vi "Process.vi"(0 "reference in":refnum<class "HPPC.lvclass">, 5 "error in":errorcluster) -> (14 "reference out":refnum<class "HPPC.lvclass">, 19 "error out":errorcluster)   [LabVIEW 2023, in "HPPC.lvclass"]
uses:
  HPPC.lvclass
  Types/DCIR Parameters.ctl
  Types/DCIR Mode.ctl
  Logger_class/Logger.lvclass
  <instrlib>/HPS-17000/HPS-17000.lvclass
  <vilib>/HPS-17000/nibatterycycler_grpc_Setpoint.ctl
  <vilib>/HPS-17000/Setpoint Stream Basic Config.ctl
  <vilib>/Utility/NIReport.llb/Report Type.ctl
  <instrlib>/HPS-17000/Internal/Set Energized Multi.vi
  <instrlib>/HPS-17000/Internal/Wait Until Energized Multi.vi
  <instrlib>/HPS-17000/Internal/Read Measurement Multi.vi
  <instrlib>/HPS-17000/Internal/Set Enabled Output Multi.vi
  <instrlib>/HPS-17000/Internal/Start Setpoint Stream Multi.vi
  <instrlib>/HPS-17000/Internal/Stream Setpoints Multi.vi
  <instrlib>/HPS-17000/Internal/Stop Setpoint Stream Multi.vi
  <instrlib>/HPS-17000/Internal/Write Setpoint Multi.vi
  <vilib>/printing/OpenHTMLReport.llb/Open HTML Report in Browser (Refnum).vi
  <vilib>/Utility/NIReport.llb/NI_report.lvclass
  HPPC.lvclass/HPPC.ctl
  <vilib>/Utility/SystemLogging/NI_SystemLogging.lvlib
  <vilib>/HPS-17000/NI_BC_client.lvlib
  <userlib>/_OpenG.lib/time/time.llb/openg_time.lvlib
  <vilib>/HPS-17000/Cycler.lvclass
  <vilib>/Utility/NIReport.llb/NI_ReportGenerationCore.lvlib
panel:
  out "Last Command":string
  out "error info":errorcluster
  in  "Save DCIR Report":bool
  in  "DCIR Tab Control":enum32{"PARAM", "PROFILE", "RUNNING", "NYQUIST"}(tab)
  out "DCIR Parameters":T1={"Initial SoC (%)"=650.0, "Pulse Mode"=2, "Pulse Current (A)"=1000.0, "Pulse Duration (S)"=500.0} {"Pulse Mode" items=["Discharge"=1, "Charge"=2]; "Initial SoC (%)" min=0.0 max=100.0}
  out "DCIR Profile":waveform(dbl)[](graph)
  out "Running Status Log":i32(listbox) caption="TEST SERVER LOG"
  out "DCIR Step":dbl[][](graph)
  out "DCIR Nyquist":cluster{dbl[], dbl[]}(graph)
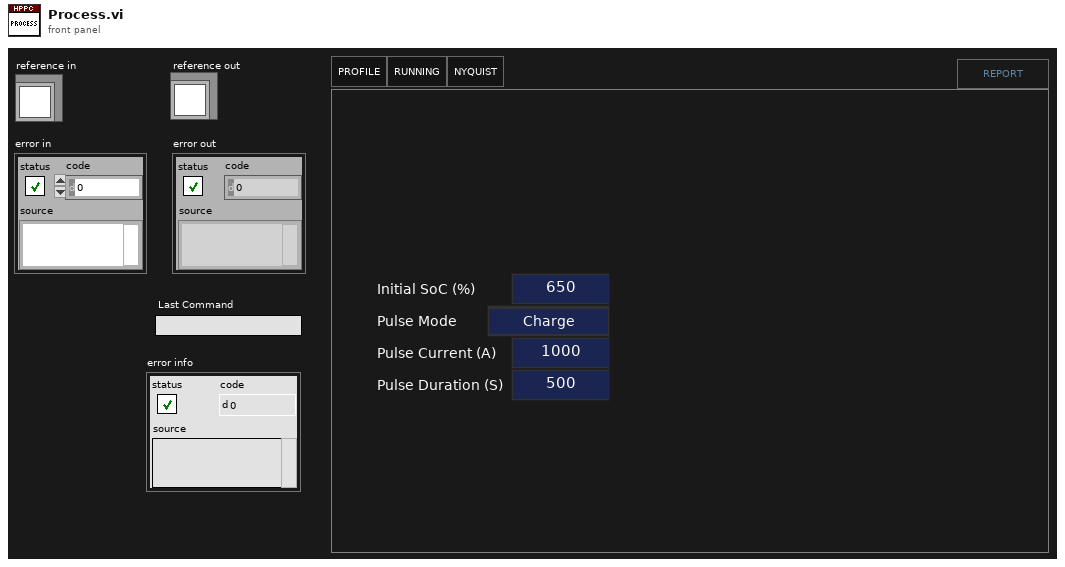
[diagram p1: front panel]
types:
  T1 = typedef "DCIR Parameters.ctl" = cluster{"Initial SoC (%)":dbl, "Pulse Mode":T2, "Pulse Current (A)":dbl, "Pulse Duration (S)":dbl}
  T2 = typedef "DCIR Mode.ctl" = u16
  T3 = cluster{"Core":cluster{"Timeout":i32, "Events":cluster{"EventsToProcess":refnum<event-registration>}, "EventFromProcess":refnum<user-event>, "ProcessSyncQueue":refnum<queue>, "QueueFromProcess":refnum<queue>, "Command":string, "Data":variant}, "DCIR Parameters":T1, "Profile Complete Event":refnum<user-event>, "DCIR Profile State":enum16{"Idle", "Start", "Run", "Stop"}, "DCIR TDMS Path":path, "Logger":refnum<class "Logger.lvclass">, "HPS17K Refs":refnum<class "HPS-17000.lvclass">[], "DCIR Profile":waveform(dbl)}
  T4 = typedef "Cycler.lvclass/Setpoint Stream Basic Config.ctl" = cluster{"local address":string, "receiver port":u16}
  T5 = typedef "NI_BC_client.lvlib/nibatterycycler_grpc_Setpoint.ctl" = cluster{"voltage":sgl, "current":sgl, "min_power":sgl, "max_power":sgl, "resistance":sgl}
  T6 = enum8{"Enabled", "Disabled", "Disabled and Grayed Out"}
  T7 = typedef "NI_ReportGenerationCore.lvlib/Report Type.ctl" = enum16{"HTML", "Word", "Excel"}
  T8 = enum32{"Invalid", "Standard", "Closed", "Hidden", "Minimized", "Maximized"}
  T9 = enum32{"PARAM", "PROFILE", "RUNNING", "NYQUIST", "PHASE", "MAGNITUDE"}
  T10 = cluster{"EventsToProcess":refnum<event-registration>}
  T11 = typedef "NI_BC_client.lvlib/MStream_grpc_CyclerMeasurement.ctl" = cluster{"measured_voltage":sgl, "measured_current":sgl, "setpoint_voltage":sgl, "setpoint_current":sgl, "timestamp":i64}
  T12 = typedef "HPPC.lvclass/ObjectAttributes.ctl" = cluster{"DCIR Parameters":T1, "Logger":refnum<class "Logger.lvclass">, "HPS17K Refs":refnum<class "HPS-17000.lvclass">[]}
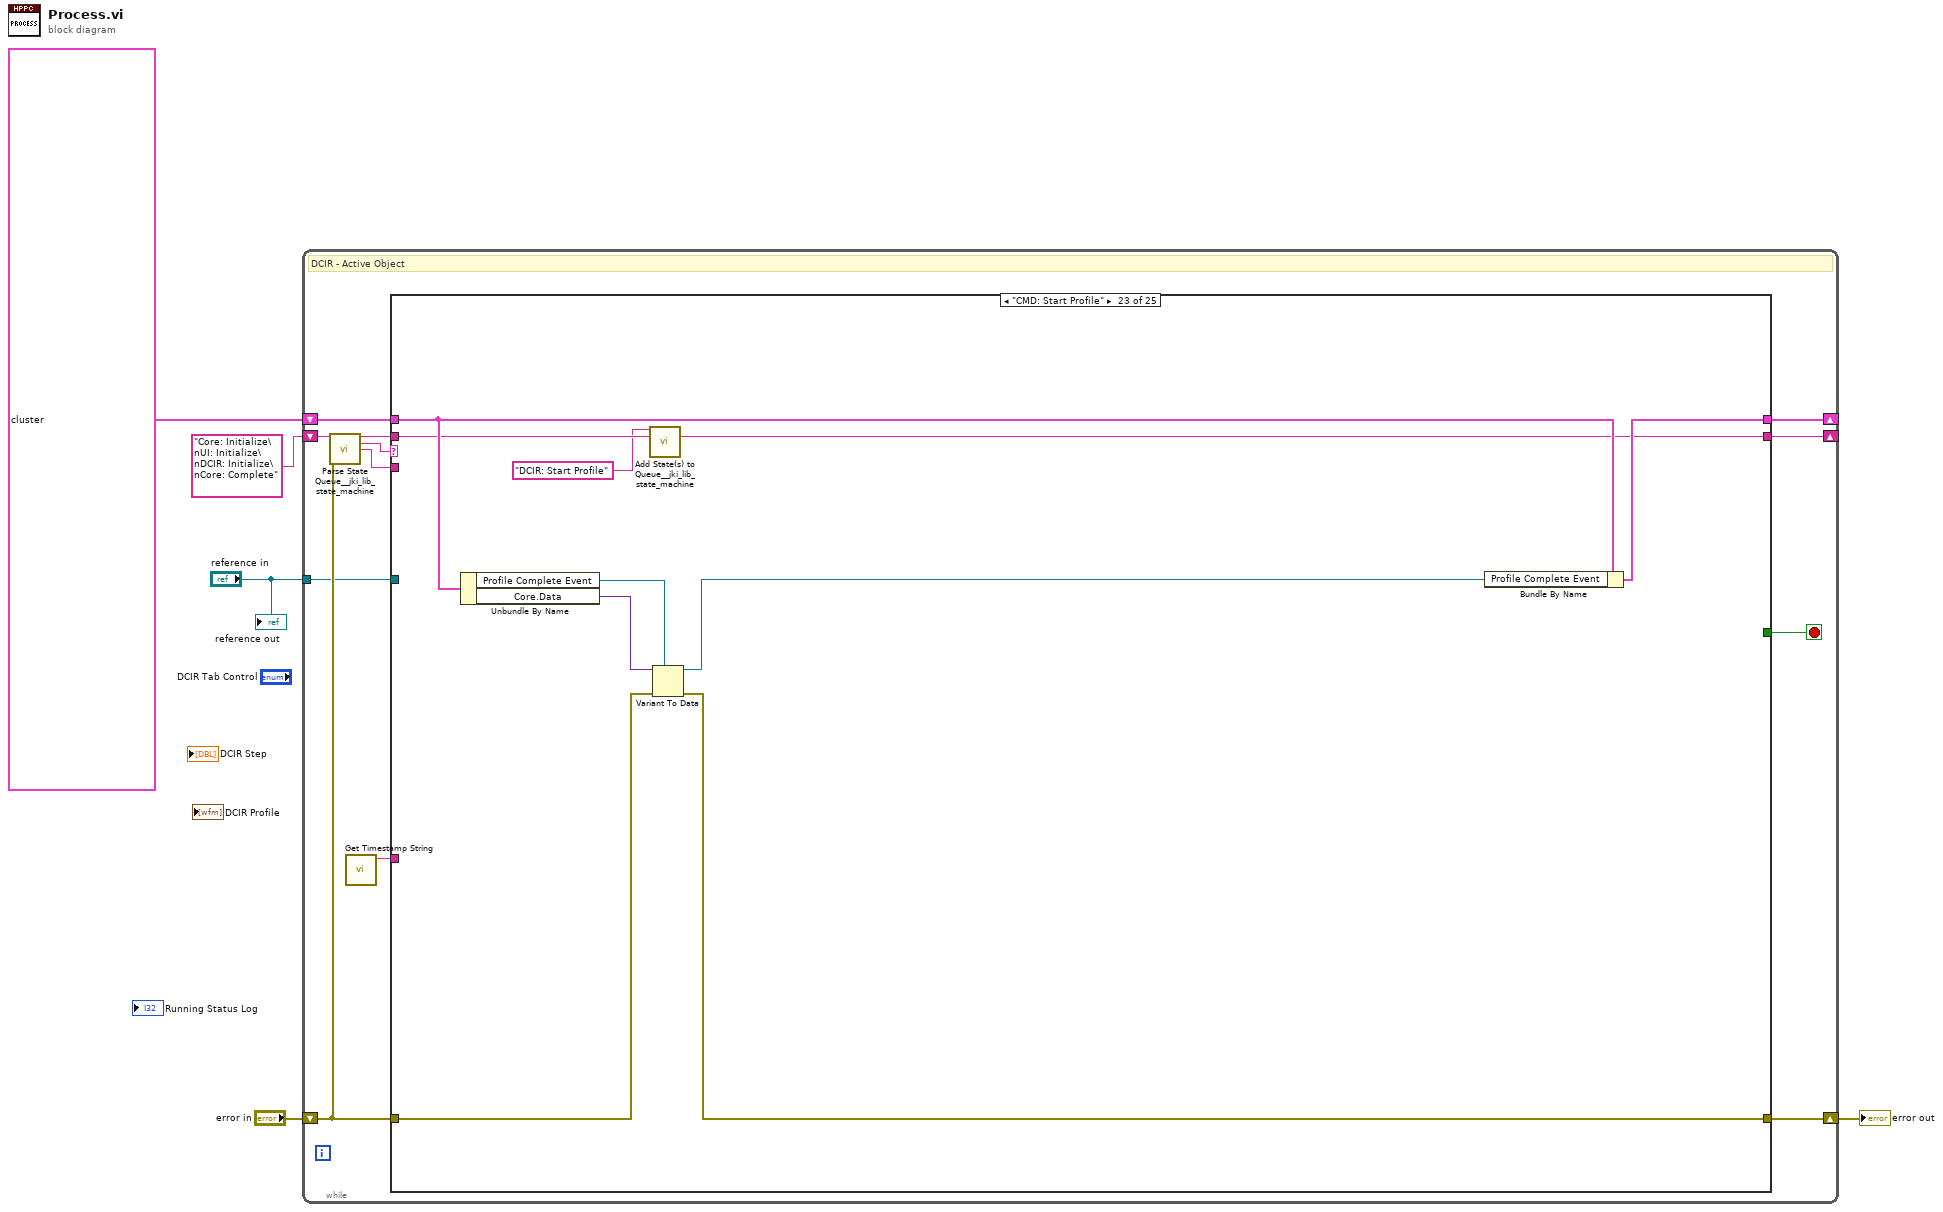
[diagram p0: block diagram]
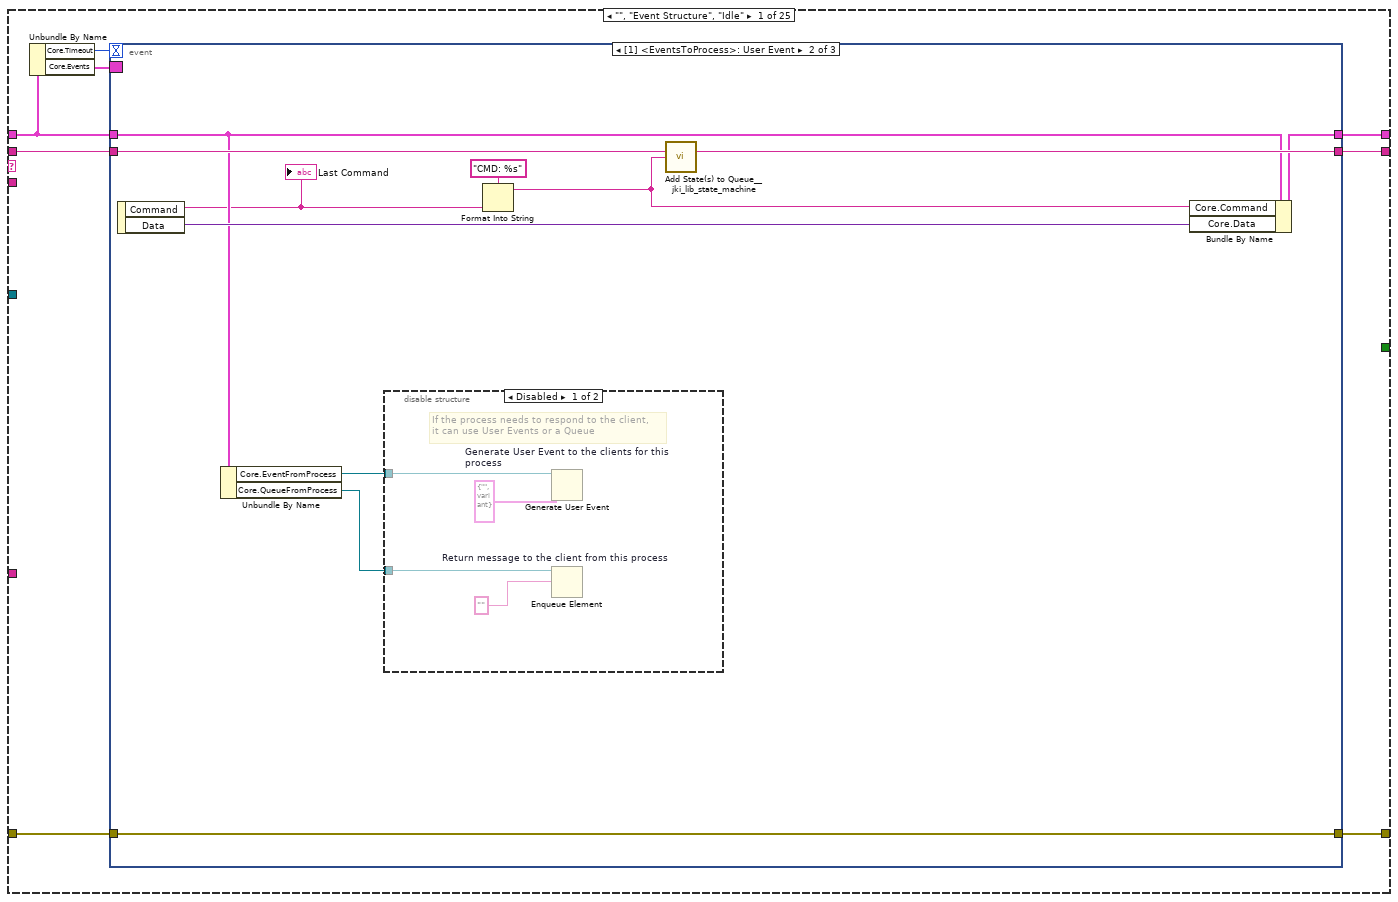
[diagram p2: hidden frame]
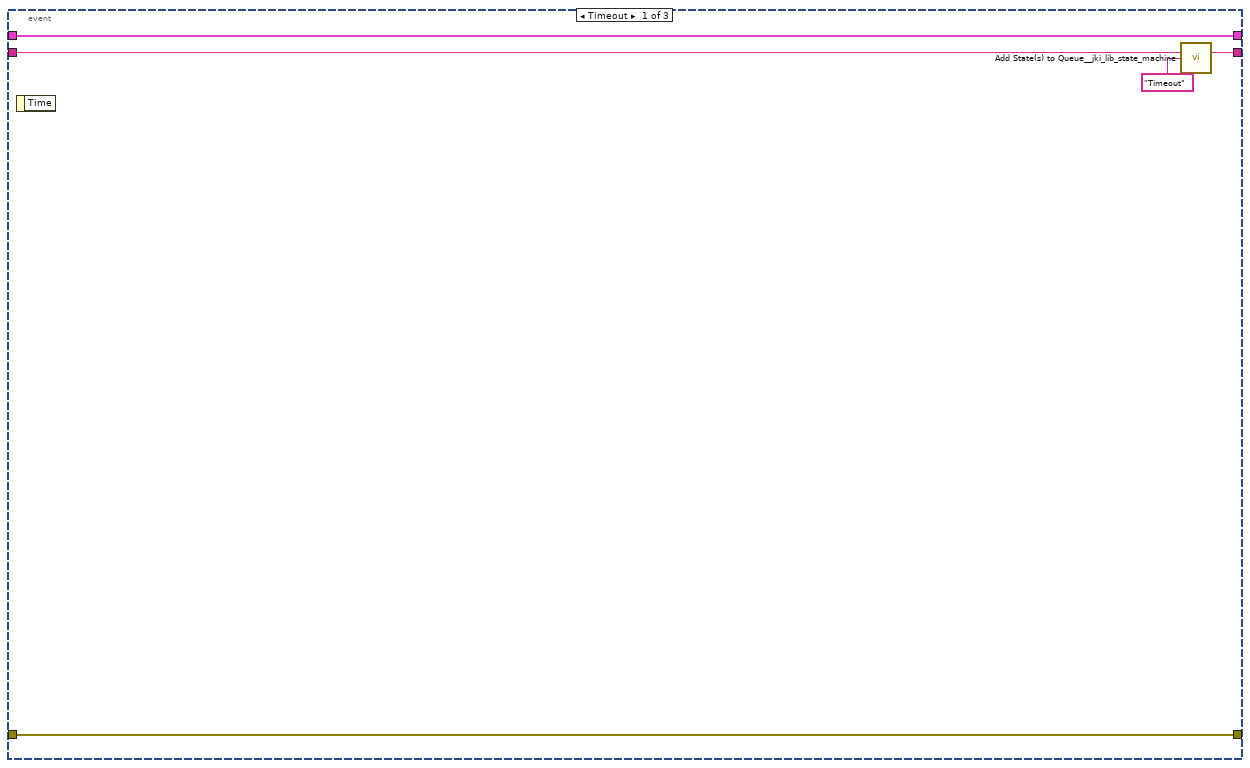
[diagram p3: hidden frame]
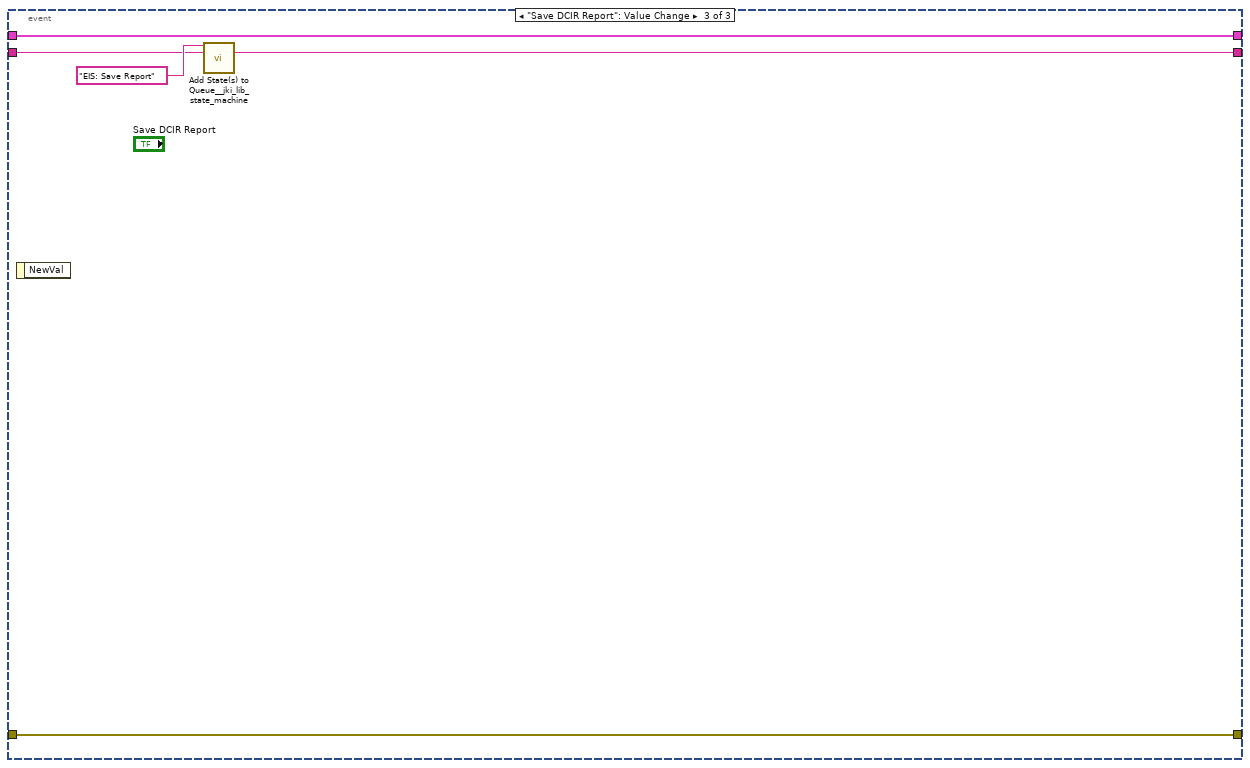
[diagram p5: hidden frame]
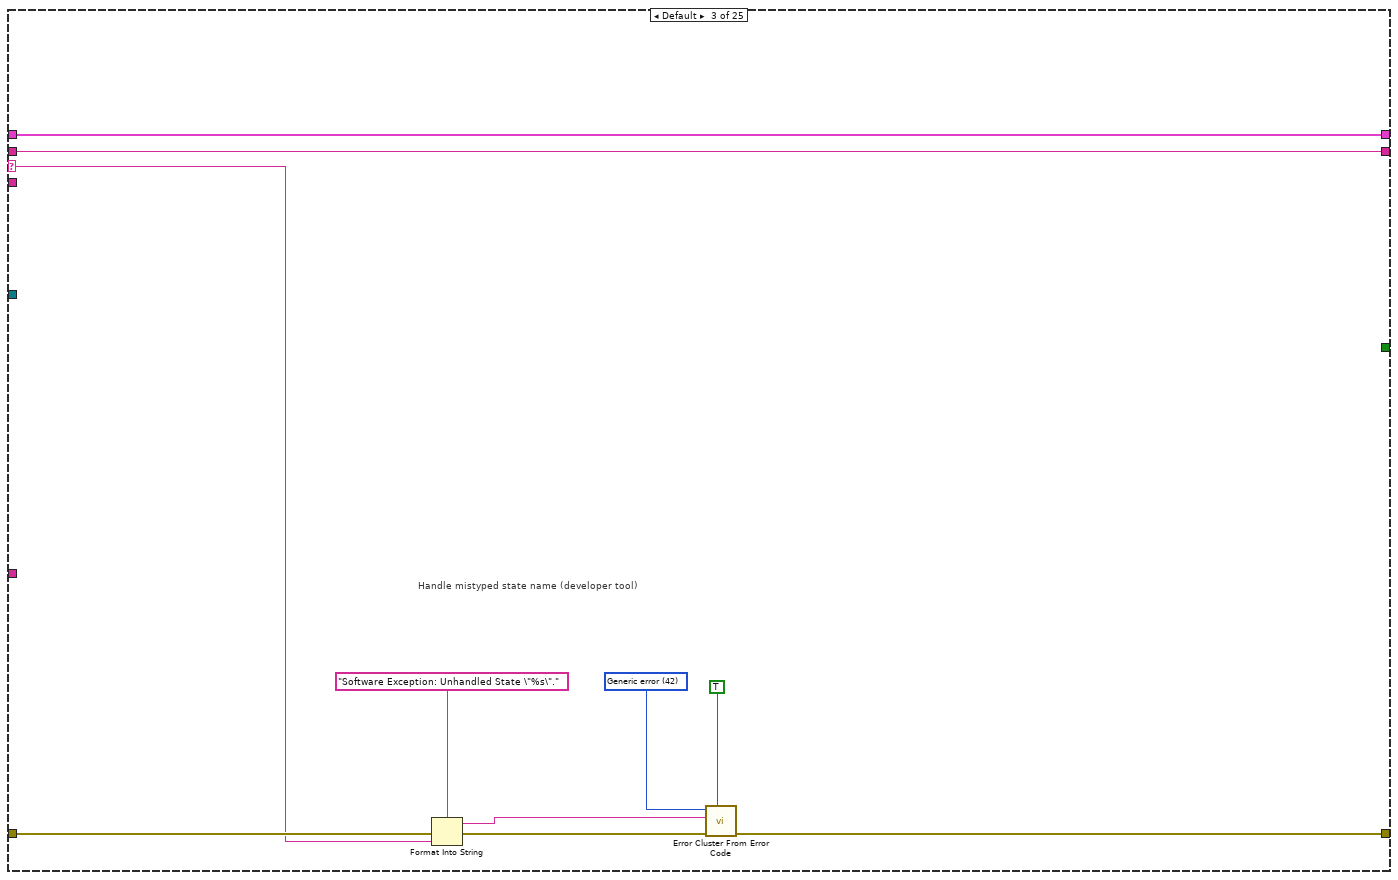
[diagram p7: hidden frame]
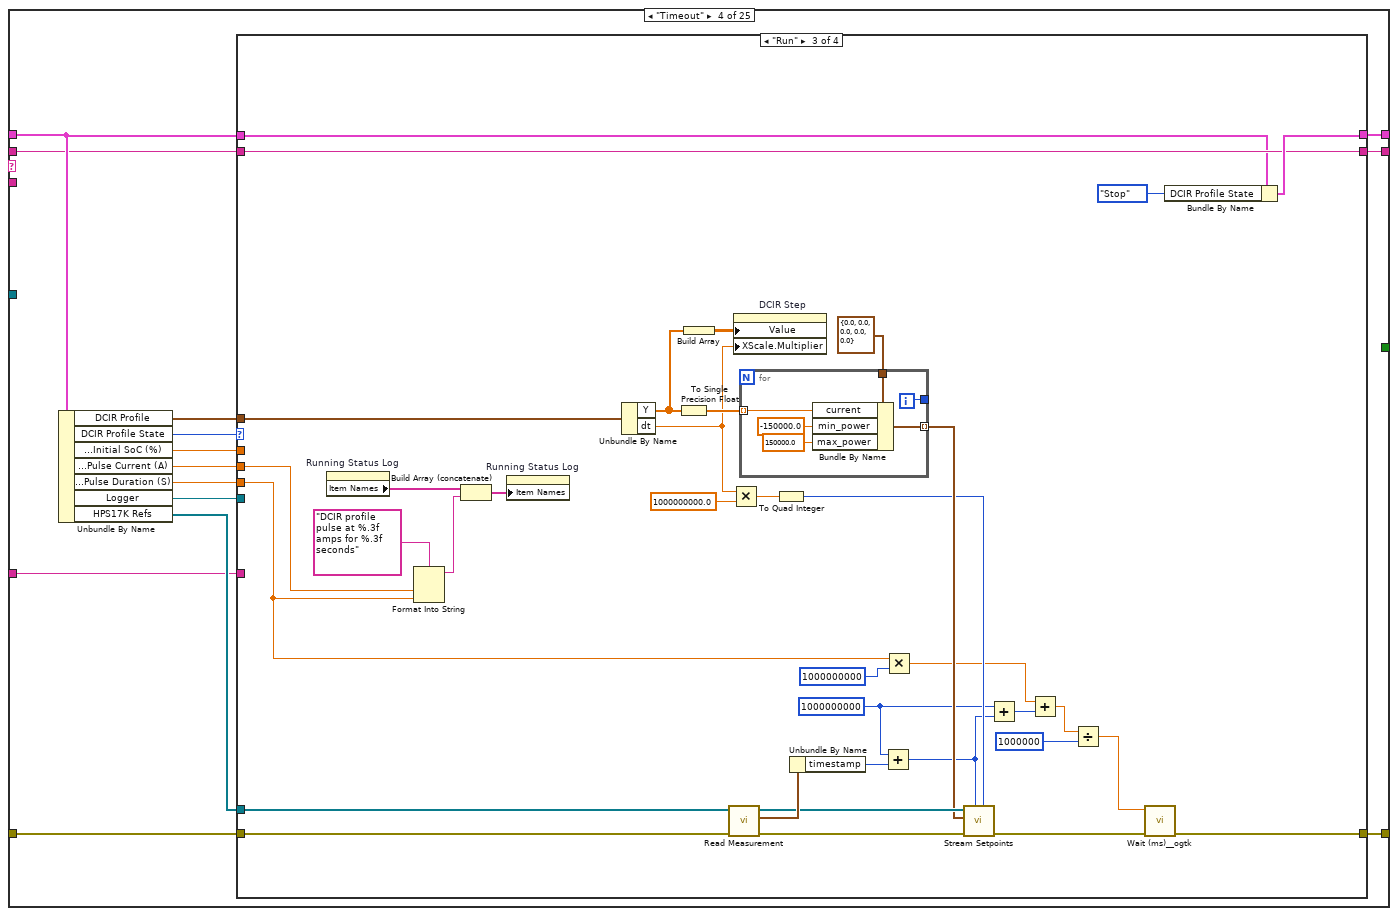
[diagram p8: hidden frame]
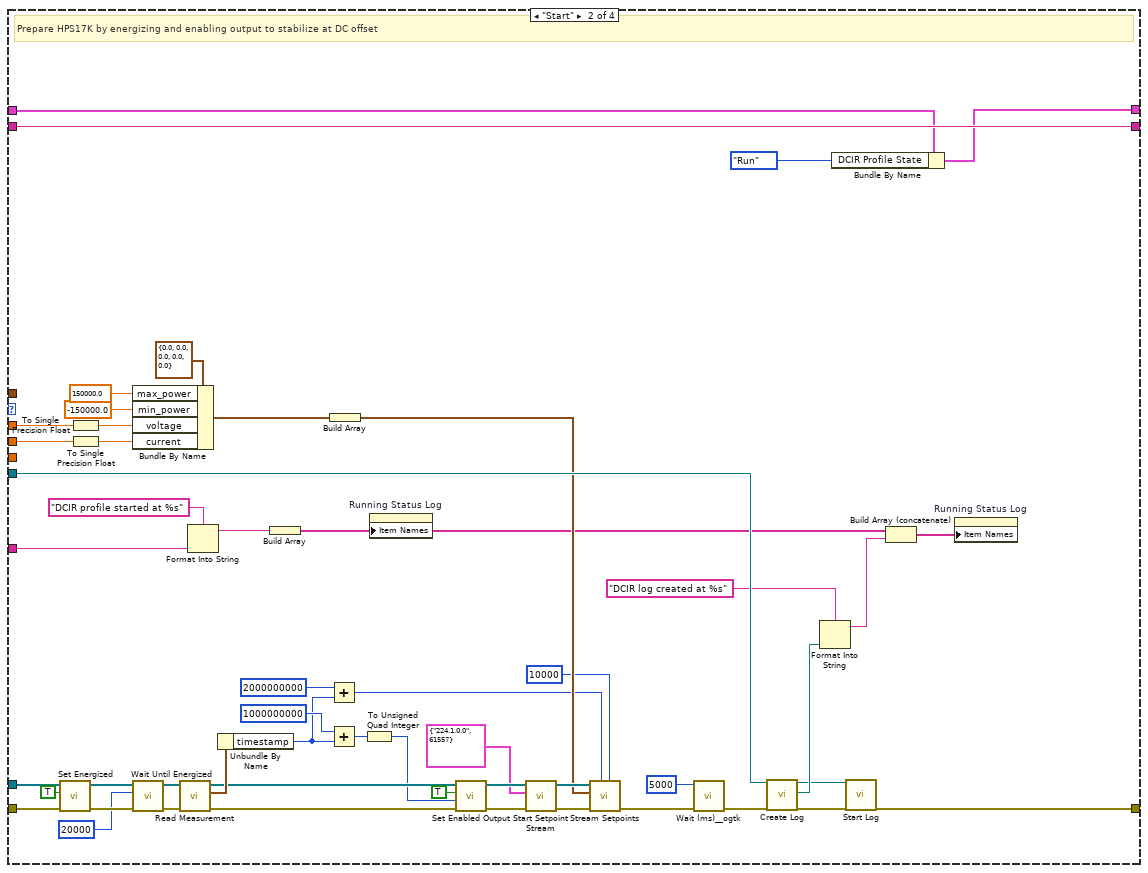
[diagram p10: hidden frame]
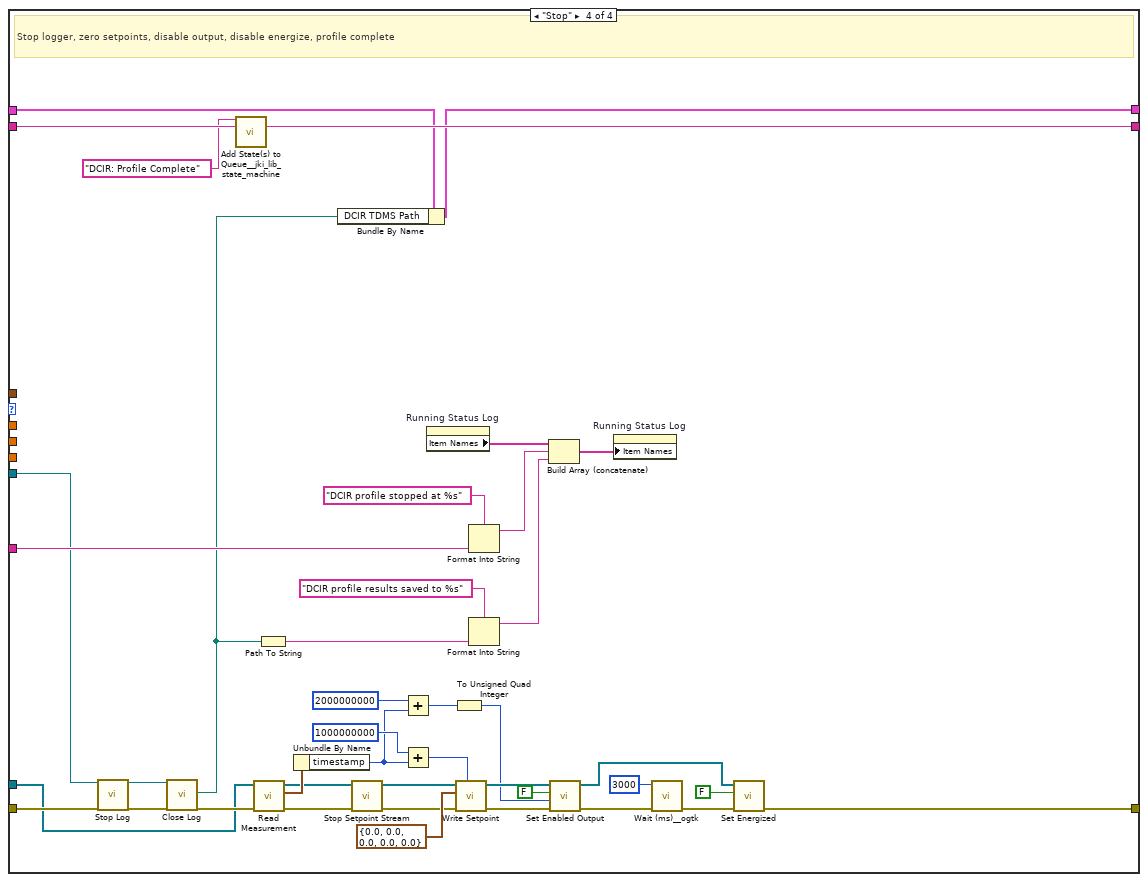
[diagram p11: hidden frame]
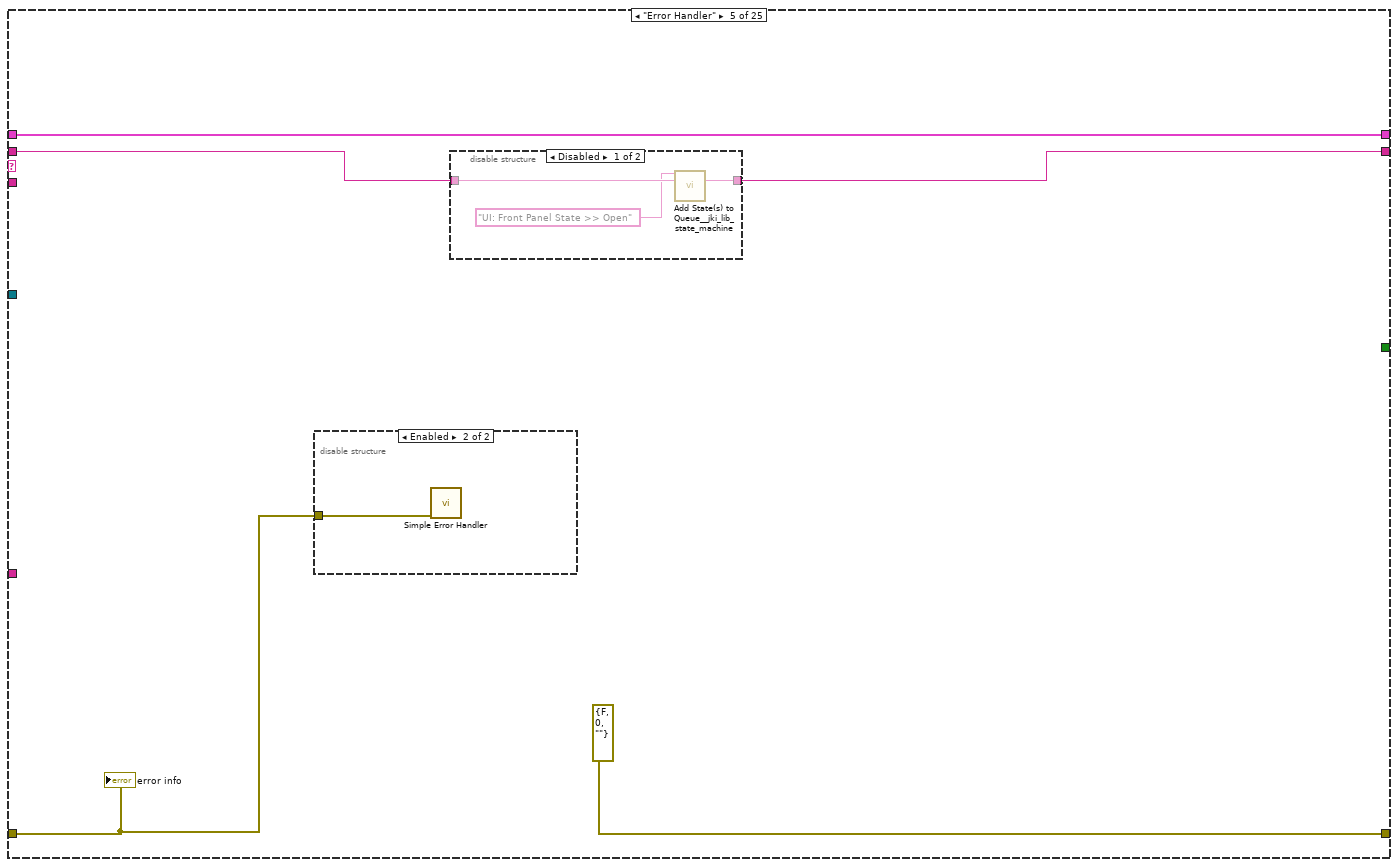
[diagram p12: hidden frame]
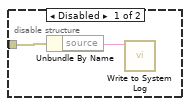
[diagram p14: hidden frame]
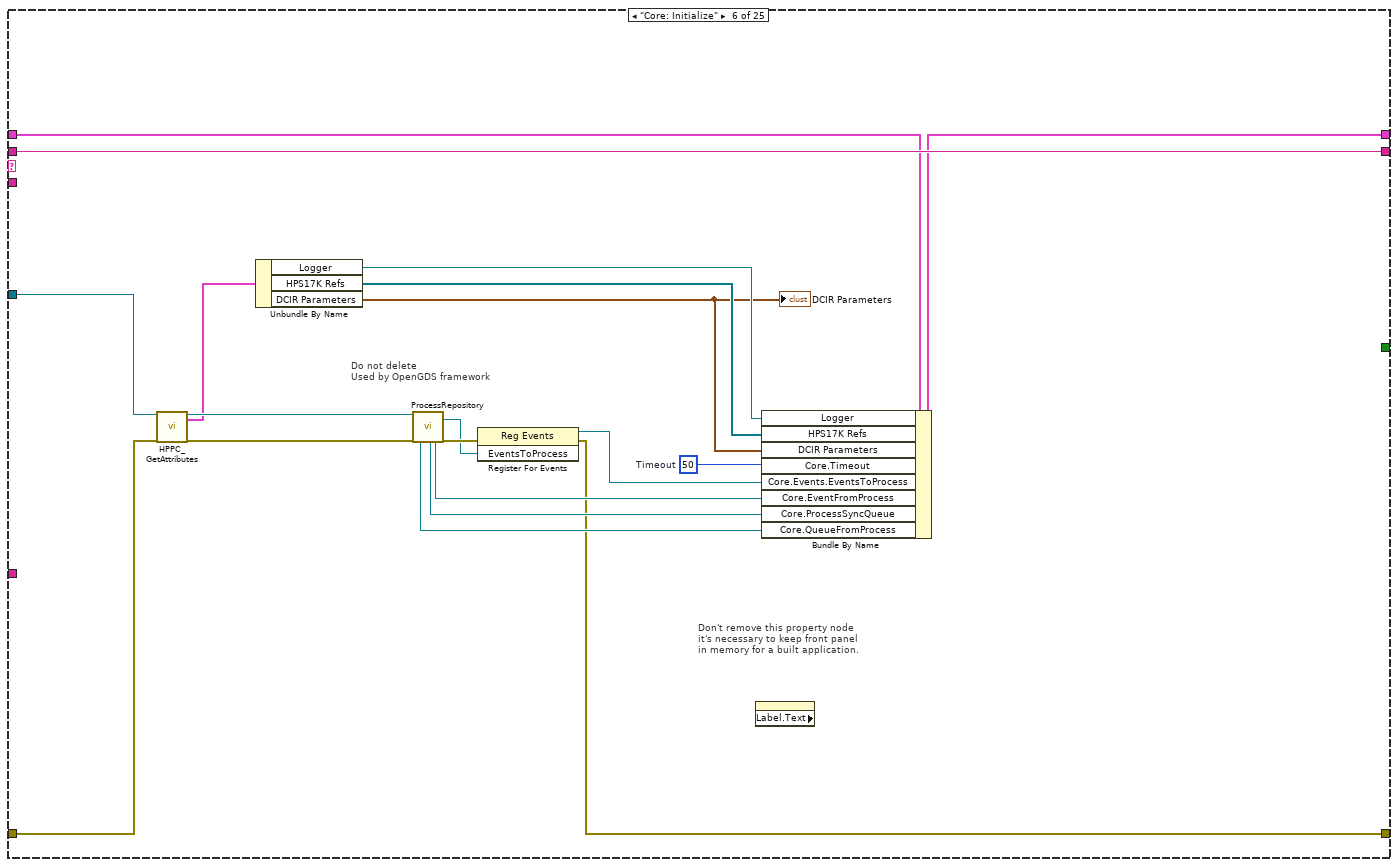
[diagram p15: hidden frame]
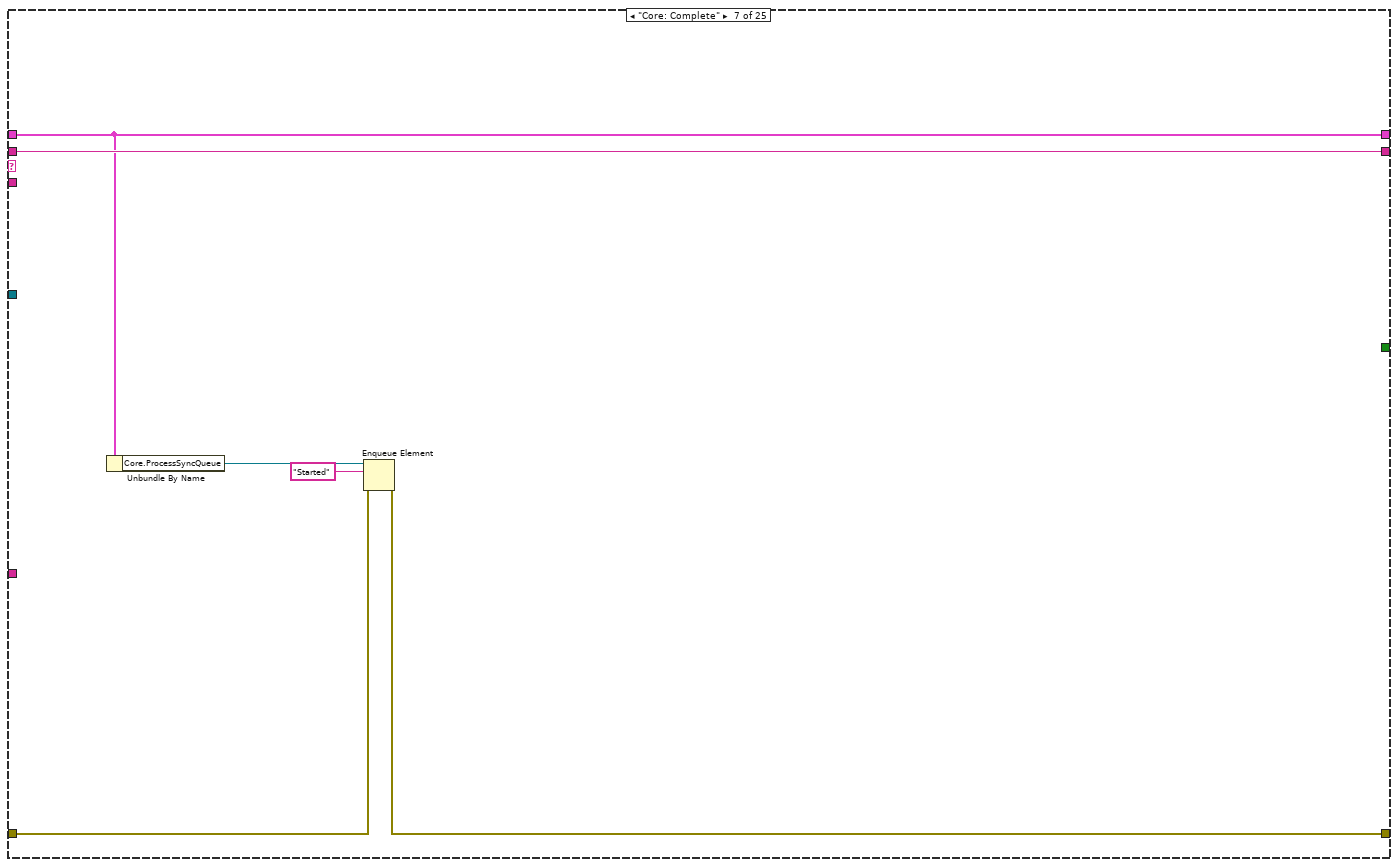
[diagram p16: hidden frame]
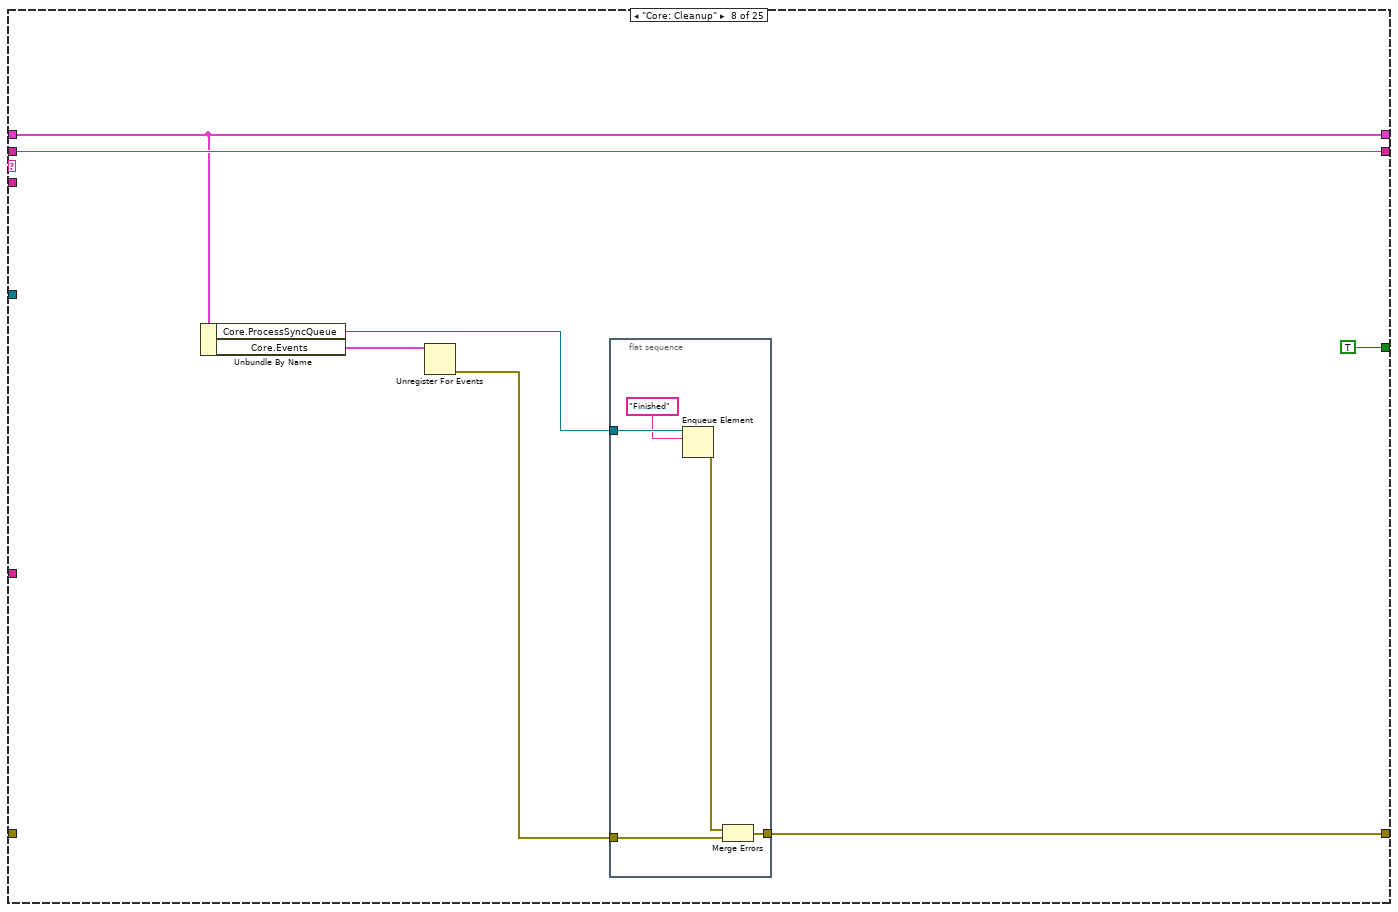
[diagram p17: hidden frame]
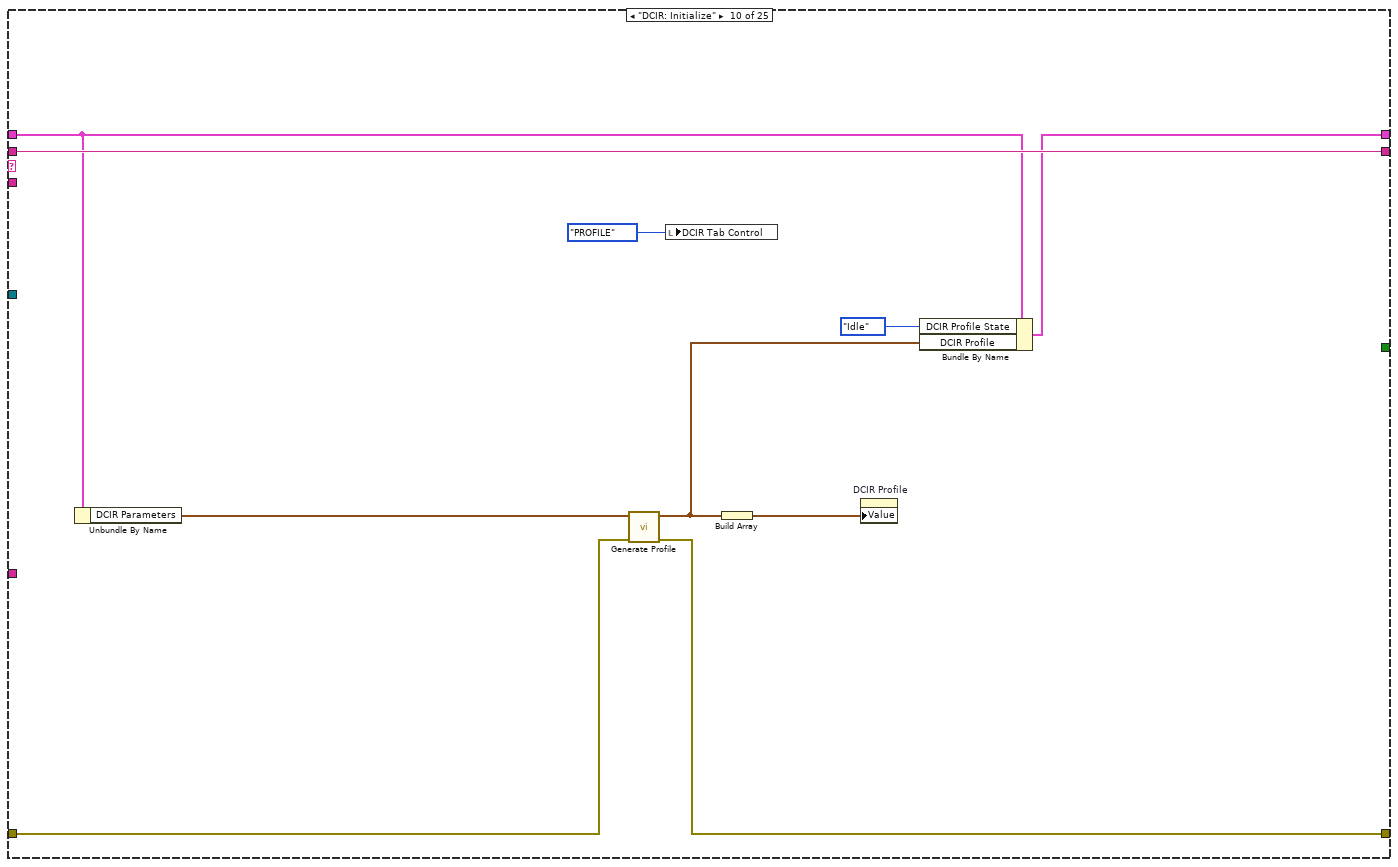
[diagram p19: hidden frame]
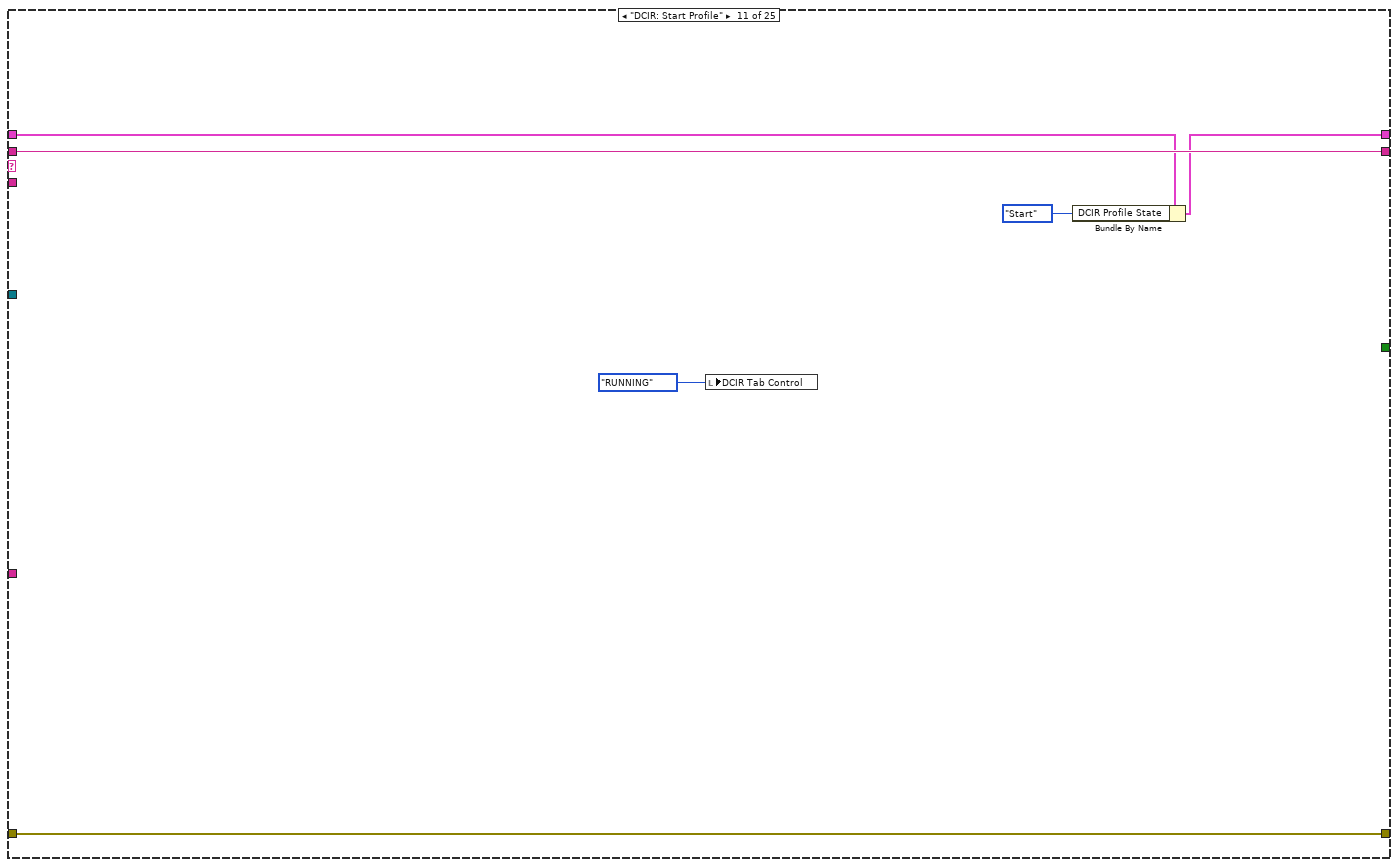
[diagram p20: hidden frame]
diagram:
  n1 = while {
    shift-right: [w16] -> w4
    shift-left: "error in" -> [w17]
    shift-right: [w9] -> _
    shift-left: "Core: Initialize\nUI: Initialize\nDCIR: Initialize\nCore: Complete" ("States Out") -> [w12]
    shift-right: [w15] -> _
    shift-left: T3 {"Core"={"Timeout"=-1, "Events"={"EventsToProcess"=refnum}, "EventFromProcess"=refnum, "ProcessSyncQueue"=refnum, "QueueFromProcess"=refnum, "Command"="", "Data"=variant}, "DCIR Parameters"={"Initial SoC (%)"=650.0, "Pulse Mode"=2, "Pulse Current (A)"=1000.0, "Pulse Duration (S)"=500.0}, "Profile Complete Event"=refnum, "DCIR Profile State"=enum."Idle", "DCIR TDMS Path"=path "", "Logger"=refnum, "HPS17K Refs"=[], "DCIR Profile"={"t0"=timestamp(0 s since 1904-01-01), "dt"=1.0, "Y"=[]}} ("LocalVariables") -> [w14]
    tunnel: "reference in" -> [w7]
    stop <- w8 stop-if-true
    # "DCIR - Active Object"
    n2 = call <vilib>:"Parse State Queue__jki_lib_state_machine.vi"("State Queue"=w12, "Error In (no error)"=w17) -> ("Remaining States"=w11:string, "Current State"=w13:string, "Arguments"=w10:string)  [unwired: 11 in]
    n3 = call "Get Timestamp String.vi"() -> ("date/time string"=w6:string)  [unwired: 11 in]
    n4 = case shown="\"CMD: Start Profile\"" w13 {
      selector: w13 -> [_ _ w54 _ _ _ _ _ _ _ _ _ _ _ _ _ _ _ _ _ _ _ _ _ _]
      tunnel: w17 -> [w19 w53 w56 w77 w217 w232 w248 _ w267 w276 w283 w288 w295 w305 w317 w364 w365 w393 _ w400 w403 w410 w418 w425 w430]
      tunnel: [w20 w53 w55 w76 errorcluster {"status"=FALSE, "code"=0, "source"=""} ("error constant") w237 w252 w255 w267 w275 w283 w288 w294 w303 w309 w364 w365 w393 w394 w400 w403 w410 w417 w425 w430] -> w16
      tunnel: [w25 w52 w63 w71 w220 w245 w249 w256 w266 w274 w280 w285 w292 w307 w319 w363 w367 w392 w395 w399 w402 w409 w415 w424 w429] -> w15
      tunnel: w14 -> [w21 w52 w63 w72 w220 w244 w249 w256 w266 w272 w281 w286 w293 w307 w319 w363 w367 w392 w395 w399 w402 w409 w416 w424 w429]
      tunnel: w11 -> [w23 w51 w62 w70 w219 w246 w251 w259 w265 w277 w282 w287 w299 w308 w318 w362 w368 w376 w397 w398 _ w408 w413 w423 w427]
      tunnel: w10 -> [_ _ _ _ _ _ _ _ _ _ _ _ _ _ _ _ w366 _ _ _ _ w405 _ _ _]
      tunnel: [w22 w51 w62 w69 w218 w246 w251 w259 w265 w277 w282 w287 w299 w308 w318 w362 w368 w376 w397 w398 "UI: Cleanup\nCore: Cleanup" ("State(s) at Back (\"\")") w407 w412 w422 w426] -> w9
      tunnel: [_ _ _ _ _ _ _ TRUE _ _ _ _ _ _ _ _ _ _ _ _ _ _ _ _ _] -> w8
      tunnel: w7 -> [_ _ _ _ _ w235 _ _ _ _ _ _ _ _ _ _ _ _ _ _ _ _ _ _ _]
      tunnel: w6 -> [_ _ _ w73 _ _ _ _ _ _ _ _ _ _ w311 _ _ _ _ _ _ _ _ _ _]
      frame "", "Event Structure", "Idle" {
        n5 = Unbundle By Name(w21) -> ("Core.Timeout"=w18:i32, "Core.Events"=w24:T10)
        n6 = event shown="[1] <EventsToProcess>: User Event" {
          selector: w24 -> [_ _ _]
          dyn-events: _ -> [_ _ _]
          timeout: w18 -> [_ _ _]
          tunnel: w21 -> [w30 w34 w50]
          tunnel: [w30 w39 w50] -> w25
          tunnel: [w28 w41 w46] -> w22
          tunnel: w23 -> [w29 w40 w47]
          tunnel: [w26 w35 w49] -> w20
          tunnel: w19 -> [w26 w35 w49]
          event Timeout {
            n7 = event-data() -> ()  [unwired: 1 in, 1 out]
            n8 = call <vilib>:"Add State(s) to Queue__jki_lib_state_machine.vi"("State(s) in (\"\")"=w29, "State(s) at Back (\"\")"="Timeout" ("State(s) at Back (\"\")")) -> ("States Out"=w28:string)  [unwired: 13 in]
          }
          event User Event {
            n9 = event-data() -> ("Command"=w32:string, "Data"=w38:variant)  [unwired: 1 in]
            "Last Command" <- w32
            n10 = Unbundle By Name(w34) -> ("Core.EventFromProcess"=w37:refnum<user-event>, "Core.QueueFromProcess"=w36:refnum<queue>)
            n11 = disable-structure shown="Disabled" {
              disable-tunnel: w37 -> [w45 _]
              disable-tunnel: w36 -> [w44 _]
              frame Disabled {
                # "If the process needs to respond to the client,\nit can use User Events or a Queue"
                n12 = Generate User Event "Generate User Event to the clients for this process"(user event=w45, event data cluster=cluster{"Command":string, "Data":variant} {"Command"="", "Data"=variant} ("event data")) -> ()  [unwired: 2 in, 2 out]
                n13 = Enqueue Element "Return message to the client from this process"(queue=w44, element="") -> ()  [unwired: 2 in, 3 out]
              }
              frame Enabled {
              }
            }
            n14 = Format Into String(format string="CMD: %s", w32) -> (resulting string=w31:string)  [unwired: 2 in, 1 out]
            n15 = call <vilib>:"Add State(s) to Queue__jki_lib_state_machine.vi"("State(s) in (\"\")"=w40, "State(s) at Back (\"\")"=w31) -> ("States Out"=w41:string)  [unwired: 13 in]
            n16 = Bundle By Name(cluster=w34, "Core.Command"=w31, "Core.Data"=w38) -> (w39:T3)
          }
          event "Save DCIR Report": Value Change {
            n17 = event-data() -> ()  [unwired: 1 in, 1 out]
            n18 = call <vilib>:"Add State(s) to Queue__jki_lib_state_machine.vi"("State(s) in Front (\"\")"="EIS: Save Report" ("State(s) in Front (\"\")"), "State(s) in (\"\")"=w47) -> ("States Out"=w46:string)  [unwired: 13 in]
          }
        }
      }
      frame "---------- Core ----------" {
      }
      frame Default {
        w60 = 42 items=["No error", "Argument error", "Memory is full", "Out of zone", "End of file", "File already open", "Generic file I/O error", "File not found", "File permission error", "Disk is full", "Duplicate path", "Too many files open", "System feature not enabled", "Resource file not found", "Cannot add resource", "Resource not found", "Image not found", "Image memory error", "Pen does not exist", "Config type invalid", "Config token not found", "Config parse error", "Config memory error", "Bad external code format", "Bad external code offset", "External code not present", "Null window", "Destroy window error", "Null menu", "Print aborted", "Bad print record", "Print driver error", "Windows error during printing", "Memory error during printing", "Print dialog error", "Generic print error", "Invalid device refnum", "Device not found", "Device parameter error", "Device unit error", "Cannot open device", "Device call aborted", "Generic error", "Cancelled by user", "Object ID too low", "Object ID too high", "Object not in heap", "Unknown heap", "Unknown object (invalid DefProc)", "Unknown object (DefProc not in table)", "Message out of range", "Invalid (null) method", "Unknown message", "Manager call not supported", "Bad address", "Network operation in progress", "Network operation timed out", "Connection is busy", "Network attribute not supported", "Network error", "Address in use", "System out of memory", "Connection aborted", "Connection refused", "Not connected", "Already connected", "Connection closed", "Initialization error (interapplication manager)", "Bad occurrence", "Wait on unbound occurrence handler", "Occurrence queue overflow", "Datalog type conflict", "Unused", "Unrecognized type (interapplication manager)", "Memory corrupt", "Failed to make temporary DLL", "Old CIN version", "Drag socket not found", "Failed to load drop-object", "Failed to register OLE object", "Failed to release OLE object", "Format specifier type mismatch", "Unknown format specifier", "Too few format specifiers", "Too many format specifiers", "Scan failed", "Newer CIN version", "Error converting to variant", "Runtime menu error", "Password tampered", "Variant attribute not found", "Incompatible variant data type", "Event data is not available", "Event Store is not present", "Occurrence is not found", "Event Queue is not created", "Event info is not available", "Refnum passed is NULL", "Error retrieving Class GUID", "Error retrieving CoClass GUID", "Error retrieving TypeLib GUID.", "Bad built application magic bytes.", "Specific driver is different from the specific driver associated with the Logical Name.", "There is no session opened to the class driver.", "Max Error", "MAX - Error with config objects", "MAX - Error loading configuration", "MAX - Group not supported"]
        # "Handle mistyped state name (developer tool)"
        n19 = Format Into String(format string="Software Exception: Unhandled State \"%s\"." ("message"), error in=w56, w54) -> (resulting string=w59:string, error out=w58:errorcluster)  [unwired: 1 in]
        n20 = call <vilib>:"Error Cluster From Error Code.vi"("show call chain? (False)"=TRUE, "error in (no error)"=w58, "error message (\"\")"=w59, "error code (0)"=w60) -> ("error out"=w55:errorcluster)  [unwired: 5 in]
      }
      frame "Timeout" {
        n21 = Unbundle By Name(w72) -> ("DCIR Profile"=w67:waveform(dbl), "DCIR Profile State"=w75:enum16{"Idle", "Start", "Run", "Stop"}, "DCIR Parameters.Initial SoC (%)"=w64:dbl, "DCIR Parameters.Pulse Current (A)"=w68:dbl, "DCIR Parameters.Pulse Duration (S)"=w65:dbl, "Logger"=w66:refnum<class "Logger.lvclass">, "HPS17K Refs"=w74:refnum<class "HPS-17000.lvclass">[])
        n22 = case shown="\"Run\"" w75 {
          tunnel: w77 -> [w80 w96 w167 w207]
          tunnel: [w80 w110 w146 w181] -> w76
          tunnel: w74 -> [_ w95 w166 w199]
          tunnel: w66 -> [_ w121 _ w204]
          tunnel: w73 -> [_ w116 _ w211]
          tunnel: w72 -> [w79 w106 w134 w180]
          tunnel: [w79 w105 w165 w179] -> w71
          tunnel: w70 -> [w78 w109 w164 w210]
          tunnel: [w78 w109 w164 w208] -> w69
          tunnel: w68 -> [_ w103 w148 _]
          tunnel: w64 -> [_ w102 _ _]
          tunnel: w67 -> [_ _ w149 _]
          tunnel: w65 -> [_ _ w137 _]
          frame "Idle", Default {
            # "do nothing"
          }
          frame "Start" {
            # "Prepare HPS17K by energizing and enabling output to stabilize at DC offset"
            n23 = call-poly <instrlib>:"Set Energized.vi"("error in"=w96, "energize (T)"=TRUE, "cycler refs in"=w95) -> ("error out"=w126:errorcluster, "cycler refs out"=w125:refnum<class "HPS-17000.lvclass">[])  [unwired: 7 in]
            n24 = To Single Precision Float(number=w102) -> (single precision float=w131:sgl)
            n25 = To Single Precision Float(number=w103) -> (single precision float=w128:sgl)
            n26 = Bundle By Name(cluster=T5 {"voltage"=0.0, "current"=0.0, "min_power"=0.0, "max_power"=0.0, "resistance"=0.0} ("setpoint"), "max_power"=sgl 150000.0, "min_power"=sgl -150000.0 ("max_power"), "voltage"=w131, "current"=w128) -> (w89:T5)
            n27 = call-poly <instrlib>:"Wait Until Energized.vi"("error in"=w126, "timeout (ms)"=u32 20000, "cycler refs in"=w125) -> ("error out"=w94:errorcluster, "cycler refs out"=w93:refnum<class "HPS-17000.lvclass">[])  [unwired: 7 in]
            n28 = call-poly <instrlib>:"Read Measurement.vi"("error in"=w94, "cycler refs in"=w93) -> ("error out"=w92:errorcluster, "aggregated cycler measurements"=w127:T11, "cycler refs out"=w91:refnum<class "HPS-17000.lvclass">[])  [unwired: 7 in]
            n29 = Format Into String(format string="DCIR profile started at %s", w116) -> (resulting string=w82:string)  [unwired: 2 in, 1 out]
            n30 = Unbundle By Name(w127) -> ("timestamp"=w97:i64)
            n31 = Build Array(w82) -> (w81:string[])
            n32 = Add(x=i64 2000000000, y=w97) -> (x+y=w86:i64)
            n33 = Add(x=i64 1000000000, y=w97) -> (x+y=w87:i64)
            n34 = Build Array(w89) -> (w88:T5[])
            n35 = To Unsigned Quad Integer(1:w87) -> (0:w85:u64)
            n36 = property on="Running Status Log" class="LstBox (strict)"("Item Names"=w81) -> ()  [unwired: 2 in, 2 out]
            n37 = call-poly <instrlib>:"Set Enabled Output.vi"("error in"=w92, "enabled timestamp"=w85, "enabled output"=TRUE, "cycler refs in"=w91) -> ("error out"=w101:errorcluster, "cycler refs out"=w100:refnum<class "HPS-17000.lvclass">[])  [unwired: 6 in]
            n38 = call-poly <instrlib>:"Start Setpoint Stream.vi"("error in"=w101, "setpoint stream config"=T4 {"local address"="224.1.0.0", "receiver port"=61557}, "cycler refs in"=w100) -> ("error out"=w98:errorcluster, "cycler refs out"=w90:refnum<class "HPS-17000.lvclass">[])  [unwired: 7 in]
            n39 = call-poly <instrlib>:"Stream Setpoints.vi"("dt"=i64 10000, "t0"=w86, "error in"=w98, "setpoints"=w88, "cycler refs in"=w90) -> ("error out"=w84:errorcluster)  [unwired: 5 in, 1 out]
            n40 = call <userlib>:"Wait (ms)__ogtk.vi"("error in (no error)"=w84, "milliseconds to wait"=u32 5000) -> ("error out"=w120:errorcluster)  [unwired: 8 in, 1 out]
            n41 = call "Create Log.vi"("reference in"=w121, "Error In"=w120) -> ("reference out"=w113:refnum<class "Logger.lvclass">, "created file"=w114:path, "Error Out"=w118:errorcluster)  [unwired: 15 in]
            n42 = Format Into String(format string="DCIR log created at %s", w114) -> (resulting string=w112:string)  [unwired: 2 in, 1 out]
            n43 = Bundle By Name(cluster=w106, "DCIR Profile State"=enum16{"Idle", "Start", "Run", "Stop"}."Run" ("EIS Profile State")) -> (w105:T3)
            n44 = call "Start Log.vi"("reference in"=w113, "Error In"=w118) -> ("Error Out"=w110:errorcluster)  [unwired: 16 in, 1 out]
            n45 = Build Array (concatenate)(w81, w112) -> (w111:string[])
            n46 = property on="Running Status Log" class="LstBox (strict)"("Item Names"=w111) -> ()  [unwired: 2 in, 2 out]
          }
          frame "Run" {
            w143 = i64 1000000000 ("x")
            n47 = property on="Running Status Log" class="LstBox (strict)"() -> ("Item Names"=w161:string[])  [unwired: 2 in, 2 out]
            n48 = Format Into String(format string="DCIR profile pulse at %.3f amps for %.3f seconds", w148, w137) -> (resulting string=w158:string)  [unwired: 2 in, 1 out]
            n49 = Build Array (concatenate)(w161, w158) -> (w157:string[])
            n50 = property on="Running Status Log" class="LstBox (strict)"("Item Names"=w157) -> ()  [unwired: 2 in, 2 out]
            n51 = Unbundle By Name(w149) -> ("Y"=w155:dbl[], "dt"=w150:dbl)
            n52 = To Single Precision Float(number=w155) -> (single precision float=w159:sgl[])
            n53 = Build Array(w155) -> (w135:dbl[][])
            n54 = call-poly <instrlib>:"Read Measurement.vi"("error in"=w167, "cycler refs in"=w166) -> ("error out"=w163:errorcluster, "aggregated cycler measurements"=w168:T11, "cycler refs out"=w162:refnum<class "HPS-17000.lvclass">[])  [unwired: 7 in]
            n55 = Multiply(x=w150, y=1000000000.0) -> (x*y=w153:dbl)
            n56 = property on="DCIR Step" class="WFGraph (strict)"("Value"=w135, "XScale.Multiplier"=w150) -> ()  [unwired: 2 in, 2 out]
            n57 = for {
              tunnel: T5 {"voltage"=0.0, "current"=0.0, "min_power"=0.0, "max_power"=0.0, "resistance"=0.0} ("nibatterycycler_grpc_Setpoint") -> [w174]
              tunnel: w159 -> [w173] mode=indexing
              tunnel: [w170] -> w152 mode=indexing
              tunnel: [w169] -> _
              i -> [w169]
              n58 = Bundle By Name(cluster=w174, "current"=w173, "min_power"=sgl -150000.0, "max_power"=sgl 150000.0) -> (w170:T5)
            }
            n59 = To Quad Integer(1:w153) -> (0:w151:i64)
            n60 = Unbundle By Name(w168) -> ("timestamp"=w133:i64)
            n61 = Add(x=w143, y=w133) -> (x+y=w144:i64)
            n62 = Multiply(x=w137, y=i64 1000000000 ("x")) -> (x*y=w136:dbl)
            n63 = call-poly <instrlib>:"Stream Setpoints.vi"("dt"=w151, "t0"=w144, "error in"=w163, "setpoints"=w152, "cycler refs in"=w162) -> ("error out"=w147:errorcluster)  [unwired: 5 in, 1 out]
            n64 = Add(x=w143, y=w144) -> (x+y=w142:i64)
            n65 = Add(x=w136, y=w142) -> (x+y=w141:dbl)
            n66 = Divide(x=w141, y=i64 1000000 ("x")) -> (x/y=w139:dbl)
            n67 = call <userlib>:"Wait (ms)__ogtk.vi"("error in (no error)"=w147, "milliseconds to wait"=w139) -> ("error out"=w146:errorcluster)  [unwired: 8 in, 1 out]
            n68 = Bundle By Name(cluster=w134, "DCIR Profile State"=enum16{"Idle", "Start", "Run", "Stop"}."Stop") -> (w165:T3)
          }
          frame "Stop" {
            # "Stop logger, zero setpoints, disable output, disable energize, profile complete"
            n69 = call "Stop Log.vi"("reference in"=w204, "Error In"=w207) -> ("reference out"=w205:refnum<class "Logger.lvclass">, "Error Out"=w206:errorcluster)  [unwired: 16 in]
            n70 = call "Close Log.vi"("reference in"=w205, "Error In"=w206) -> ("log file path"=w175:path, "Error Out"=w200:errorcluster)  [unwired: 15 in, 1 out]
            n71 = call <vilib>:"Add State(s) to Queue__jki_lib_state_machine.vi"("State(s) in Front (\"\")"="DCIR: Profile Complete" ("State(s) in Front (\"\")"), "State(s) in (\"\")"=w210) -> ("States Out"=w208:string)  [unwired: 13 in]
            n72 = call-poly <instrlib>:"Read Measurement.vi"("error in"=w200, "cycler refs in"=w199) -> ("error out"=w185:errorcluster, "aggregated cycler measurements"=w203:T11, "cycler refs out"=w184:refnum<class "HPS-17000.lvclass">[])  [unwired: 7 in]
            n73 = Path To String(path=w175) -> (string=w177:string)
            n74 = Unbundle By Name(w203) -> ("timestamp"=w194:i64)
            n75 = Bundle By Name(cluster=w180, "DCIR TDMS Path"=w175) -> (w179:T3)
            n76 = call-poly <instrlib>:"Stop Setpoint Stream.vi"("error in"=w185, "cycler refs in"=w184) -> ("error out"=w183:errorcluster, "cycler refs out"=w182:refnum<class "HPS-17000.lvclass">[])  [unwired: 8 in]
            n77 = Add(x=i64 2000000000, y=w194) -> (x+y=w195:i64)
            n78 = Add(x=i64 1000000000, y=w194) -> (x+y=w202:i64)
            n79 = property on="Running Status Log" class="LstBox (strict)"() -> ("Item Names"=w215:string[])  [unwired: 2 in, 2 out]
            n80 = To Unsigned Quad Integer(1:w195) -> (0:w191:u64)
            n81 = call-poly <instrlib>:"Write Setpoint.vi"("timestamp"=w202, "error in"=w183, "setpoint"=T5 {"voltage"=0.0, "current"=0.0, "min_power"=0.0, "max_power"=0.0, "resistance"=0.0}, "cycler refs in"=w182) -> ("error out"=w193:errorcluster, "cycler refs out"=w192:refnum<class "HPS-17000.lvclass">[])  [unwired: 6 in]
            n82 = Format Into String(format string="DCIR profile stopped at %s", w211) -> (resulting string=w214:string)  [unwired: 2 in, 1 out]
            n83 = Format Into String(format string="DCIR profile results saved to %s", w177) -> (resulting string=w176:string)  [unwired: 2 in, 1 out]
            n84 = Build Array (concatenate)(w215, w214, w176) -> (w213:string[])
            n85 = call-poly <instrlib>:"Set Enabled Output.vi"("error in"=w193, "enabled timestamp"=w191, "enabled output"=FALSE, "cycler refs in"=w192) -> ("error out"=w189:errorcluster, "cycler refs out"=w187:refnum<class "HPS-17000.lvclass">[])  [unwired: 6 in]
            n86 = property on="Running Status Log" class="LstBox (strict)"("Item Names"=w213) -> ()  [unwired: 2 in, 2 out]
            n87 = call <userlib>:"Wait (ms)__ogtk.vi"("error in (no error)"=w189, "milliseconds to wait"=u32 3000) -> ("error out"=w188:errorcluster)  [unwired: 8 in, 1 out]
            n88 = call-poly <instrlib>:"Set Energized.vi"("error in"=w188, "energize (T)"=FALSE, "cycler refs in"=w187) -> ("error out"=w181:errorcluster)  [unwired: 7 in, 1 out]
          }
        }
      }
      frame "Error Handler" {
        n89 = disable-structure shown="Enabled" {
          disable-tunnel: w217 -> [w226 w227]
          frame Disabled {
            n90 = Unbundle By Name(w226) -> ("source"=w225:string)
            n91 = call <vilib>:"Write to System Log.vi"("message"=w225) -> ()  [unwired: 10 in, 1 out]
          }
          frame Enabled {
            n92 = call <vilib>:"Simple Error Handler.vi"("error in (no error)"=w227) -> ()  [unwired: 4 in, 5 out]
          }
        }
        n93 = disable-structure shown="Disabled" {
          disable-tunnel: w219 -> [w223 w224]
          disable-tunnel: [w222 w224] -> w218
          frame Disabled {
            n94 = call <vilib>:"Add State(s) to Queue__jki_lib_state_machine.vi"("State(s) in Front (\"\")"="UI: Front Panel State >> Open" ("State(s) at Back (\"\")"), "State(s) in (\"\")"=w223) -> ("States Out"=w222:string)  [unwired: 13 in]
          }
          frame Enabled {
          }
        }
        "error info" <- w217
      }
      frame "Core: Initialize" {
        w236 = 50  # Timeout
        # "Do not delete\nUsed by OpenGDS framework"
        # "Don't remove this property node\nit's necessary to keep front panel\nin memory for a built application."
        # "Template created by VI Technologies"
        n95 = call "HPPC_GetAttributes.vi"("reference in"=w235, "Error In"=w232) -> ("reference out"=w234:refnum<class "HPPC.lvclass">, "Data"=w231:T12, "Error Out"=w233:errorcluster)  [unwired: 14 in, 1 out]
        n96 = Unbundle By Name(w231) -> ("Logger"=w229:refnum<class "Logger.lvclass">, "HPS17K Refs"=w230:refnum<class "HPS-17000.lvclass">[], "DCIR Parameters"=w228:T1)
        "DCIR Parameters" <- w228
        n97 = call "ProcessRepository.vi"("reference in"=w234, "Error In"=w233) -> ("QueueFromProcess"=w239:refnum<queue>, "ProcessSyncQueue"=w238:refnum<queue>, "EventFromProcess"=w240:refnum<user-event>, "EventsToProcess"=w242:refnum<user-event>, "Error Out"=w243:errorcluster)  [unwired: 10 in, 3 out]
        n98 = register-events(error in=w243, w242) -> (reference out=w241:refnum<event-registration>, error out=w237:errorcluster)  [unwired: 1 in]
        n99 = property on="reference in" class="LVClassControl (strict)" props=["Label", "Text"]() -> ()  [unwired: 2 in, 3 out]
        n100 = Bundle By Name(cluster=w244, "Logger"=w229, "HPS17K Refs"=w230, "DCIR Parameters"=w228, "Core.Timeout"=w236, "Core.Events.EventsToProcess"=w241, "Core.EventFromProcess"=w240, "Core.ProcessSyncQueue"=w238, "Core.QueueFromProcess"=w239) -> (w245:T3)
      }
      frame "Core: Complete" {
        # "Template created by VI Technologies"
        n101 = Unbundle By Name(w249) -> ("Core.ProcessSyncQueue"=w247:refnum<queue>)
        n102 = Enqueue Element(queue=w247, element="Started", error in (no error)=w248) -> (error out=w252:errorcluster)  [unwired: 1 in, 2 out]
      }
      frame "Core: Cleanup" {
        n103 = Unbundle By Name(w256) -> ("Core.ProcessSyncQueue"=w257:refnum<queue>, "Core.Events"=w254:T10)
        n104 = Unregister For Events(event registration refnum=w254) -> (error out=w253:errorcluster)  [unwired: 1 in]
        n105 = flat-sequence {
          tunnel: [w263] -> w255
          tunnel: w257 -> [w262]
          tunnel: w253 -> [w261]
          frame #0 {
            n106 = Enqueue Element(queue=w262, element="Finished") -> (error out=w264:errorcluster)  [unwired: 2 in, 2 out]
            n107 = Merge Errors(w264, w261) -> (w263:errorcluster)
          }
        }
      }
      frame "---------- DCIR ----------" {
      }
      frame "DCIR: Initialize" {
        n108 = Unbundle By Name(w272) -> ("DCIR Parameters"=w268:T1)
        n109 = call "Generate Profile.vi"("error in (no error)"=w276, "DCIR Parameters"=w268) -> ("error out"=w275:errorcluster, "DCIR Profile"=w270:waveform(dbl))  [unwired: 8 in]
        n110 = local write "DCIR Tab Control"(enum32{"PARAM", "PROFILE", "RUNNING", "NYQUIST"}."PROFILE" ("EIS Tab Control")) -> ()
        n111 = Build Array(w270) -> (w269:waveform(dbl)[])
        n112 = property on="DCIR Profile" class="WFGraph (strict)"("Value"=w269) -> ()  [unwired: 2 in, 2 out]
        n113 = Bundle By Name(cluster=w272, "DCIR Profile State"=enum16{"Idle", "Start", "Run", "Stop"}."Idle" ("EIS Profile State"), "DCIR Profile"=w270) -> (w274:T3)
      }
      frame "DCIR: Start Profile" {
        n114 = local write "DCIR Tab Control"(enum32{"PARAM", "PROFILE", "RUNNING", "NYQUIST"}."RUNNING" ("EIS Tab Control")) -> ()
        n115 = Bundle By Name(cluster=w281, "DCIR Profile State"=enum16{"Idle", "Start", "Run", "Stop"}."Start" ("EIS Profile State")) -> (w280:T3)
      }
      frame "DCIR: Stop Profile" {
        n116 = Bundle By Name(cluster=w286, "DCIR Profile State"=enum16{"Idle", "Start", "Run", "Stop"}."Stop" ("EIS Profile State")) -> (w285:T3)
      }
      frame "DCIR: Profile Complete" {
        n117 = Unbundle By Name(w293) -> ("Profile Complete Event"=w298:refnum<user-event>, "DCIR TDMS Path"=w291:path)
        n118 = Path To String(path=w291) -> (string=w290:string)
        n119 = Format Into String(format string="DCIR Profile data saved to %s" ("event data"), w290) -> (resulting string=w296:string)  [unwired: 2 in, 1 out]
        n120 = Generate User Event(user event=w298, event data cluster=w296, error in=w295) -> (error out=w294:errorcluster)  [unwired: 1 in, 1 out]
        n121 = Bundle By Name(cluster=w293, "DCIR Profile State"=enum16{"Idle", "Start", "Run", "Stop"}."Idle" ("EIS Profile State")) -> (w292:T3)
      }
      frame "DCIR: Generate Plots" {
        n122 = Unbundle By Name(w307) -> ("DCIR TDMS Path"=w306:path, "DCIR Parameters"=w300:T1)
        n123 = call "Generate DCIR Plots.vi"("error in (no error)"=w305, "DCIR Parameters"=w300, "TDMS Data File"=w306) -> ("error out"=w303:errorcluster, "DCIR Nyquist"=→"DCIR Nyquist":cluster{dbl[], dbl[]})  [unwired: 7 in]
        n124 = local write "DCIR Tab Control"(enum32{"PARAM", "PROFILE", "RUNNING", "NYQUIST"}."NYQUIST" ("EIS Tab Control")) -> ()
        n125 = property on="Save DCIR Report" class="Bool"("DisabledEnum"=T6."Enabled" ("Disabled")) -> ()  [unwired: 2 in, 2 out]
      }
      frame "DCIR: Save Report" {
        n126 = call "File Dialog"("error in"=w317, "pattern (all files)"="*.html", "pattern label"="HTML Report") -> ("selected path"=w310:path, "cancelled"=w314:bool, "error out"=w312:errorcluster)  [unwired: 9 in, 1 out]
        n127 = Or(x=w314, y=w312) -> (x .or. y?=w313:bool)
        n128 = case shown="False" w313 {
          tunnel: w312 -> [w359 w361]
          tunnel: w311 -> [w354 _]
          tunnel: w310 -> [w351 _]
          tunnel: [w345 w361] -> w309
          frame False {
            w349 = enum16{".jpg", ".png"}.".png" ("image file type (.jpg)")
            # "#TODO"
            n129 = property on="Running Status Log" class="LstBox (strict)"() -> ("Item Names"=w348:string[])  [unwired: 2 in, 2 out]
            n130 = call <vilib>:"Create Report.vi"("report type"=Report_Type."HTML", "error in (no error)"=w359) -> ("report out"=w357:refnum<class "NI_report.lvclass">, "error out"=w358:errorcluster)  [unwired: 12 in]
            n131 = call-dynamic "Set Report Header Text.vi"("report in"=w357, "left header text"="HPS17K Panel", "center header text"="DCIR Report", "right header text"=w354, "error in (no error)"=w358) -> ("report out"=w336:refnum<class "NI_report.lvclass">, "error out"=w337:errorcluster)  [unwired: 9 in]
            n132 = call-dynamic "Append Horizontal Line to Report.vi"("report in"=w336, "error in (no error)"=w337) -> ("report out"=w334:refnum<class "NI_report.lvclass">, "error out"=w335:errorcluster)  [unwired: 12 in]
            n133 = control-ref of="DCIR Profile"() -> (w344:refnum<vi>)
            n134 = call-dynamic "Append List to Report.vi"("report in"=w334, "list elements"=w348, "error in (no error)"=w335) -> ("report out"=w332:refnum<class "NI_report.lvclass">, "error out"=w333:errorcluster)  [unwired: 9 in, 2 out]
            n135 = control-ref of="DCIR Nyquist"() -> (w352:refnum<vi>)
            n136 = control-ref of="DCIR Parameters"() -> (w338:refnum<vi>)
            n137 = call-dynamic "Append Horizontal Line to Report.vi"("report in"=w332, "error in (no error)"=w333) -> ("report out"=w330:refnum<class "NI_report.lvclass">, "error out"=w331:errorcluster)  [unwired: 12 in]
            n138 = call-dynamic "Append Control Image to Report.vi"("report in"=w330, "ctrl reference"=w338, "description"="DCIR Parameters", "error in (no error)"=w331) -> ("report out"=w328:refnum<class "NI_report.lvclass">, "error out"=w329:errorcluster)  [unwired: 8 in, 2 out]
            n139 = call-dynamic "Append Horizontal Line to Report.vi"("report in"=w328, "error in (no error)"=w329) -> ("report out"=w326:refnum<class "NI_report.lvclass">, "error out"=w327:errorcluster)  [unwired: 12 in]
            n140 = call-dynamic "Append Control Image to Report.vi"("report in"=w326, "image file type (.jpg)"=w349, "ctrl reference"=w344, "description"="DCIR Profile", "error in (no error)"=w327) -> ("report out"=w324:refnum<class "NI_report.lvclass">, "error out"=w325:errorcluster)  [unwired: 7 in, 2 out]
            n141 = call-dynamic "Append Horizontal Line to Report.vi"("report in"=w324, "error in (no error)"=w325) -> ("report out"=w322:refnum<class "NI_report.lvclass">, "error out"=w323:errorcluster)  [unwired: 12 in]
            n142 = call-dynamic "Append Control Image to Report.vi"("report in"=w322, "image file type (.jpg)"=w349, "ctrl reference"=w352, "description"="DCIR Nyquist", "error in (no error)"=w323) -> ("report out"=w321:refnum<class "NI_report.lvclass">, "error out"=w320:errorcluster)  [unwired: 7 in, 2 out]
            n143 = call-dynamic "Append User Formatted HTML to Report.vi"("report in"=w321, "HTML text"="<style>body {background-color:#111111;color:#ECECED}</style>", "error in (no error)"=w320) -> ("report out"=w342:refnum<class "NI_report.lvclass">, "error out"=w343:errorcluster)  [unwired: 11 in]
            n144 = call-dynamic "Save Report to File.vi"("report in"=w342, "report file path"=w351, "prompt to replace? (F)"=TRUE, "error in (no error)"=w343) -> ("report out"=w347:refnum<class "NI_report.lvclass">, "error out"=w346:errorcluster)  [unwired: 10 in]
            n145 = call-poly <vilib>:"Open HTML Report in Browser.vi"("report in"=w347, "error in (no error)"=w346) -> ("error out"=w345:errorcluster)  [unwired: 11 in, 2 out]
          }
          frame True {
          }
        }
      }
      frame "---------- UI ----------" {
      }
      frame "UI: Front Panel State" {
        n146 = case shown="\"Close\"" w366 {
          frame "Open", Default {
            n147 = property class="VI"() -> ("FP.State"=w369:T8)  [unwired: 2 in, 2 out]
            n148 = case shown="Default" w369 {
              frame Default {
                n149 = invoke class="VI" method="FP.Open"("Activate"=TRUE, "State"=T8."Standard") -> ()  [unwired: 3 in, 5 out]
              }
              frame "Standard" {
              }
            }
          }
          frame "Close" {
            n150 = property class="VI"() -> ("FP.State"=w372:T8)  [unwired: 2 in, 2 out]
            n151 = case shown="Default" w372 {
              frame "Closed" {
              }
              frame Default {
                n152 = invoke class="VI" method="FP.Close"() -> ()  [unwired: 3 in, 3 out]
              }
            }
          }
        }
      }
      frame "UI: Initialize" {
        n153 = property class="VI"() -> ("Name"=w389:string)  [unwired: 2 in, 2 out]
        n154 = Match Pattern(string=w389, regular expression="\\2Evi$") -> (before substring=w387:string)  [unwired: 1 in, 3 out]
        n155 = local write "DCIR Tab Control"(T9."PROFILE" ("EIS Tab Control")) -> ()
        n156 = property on="Running Status Log" class="LstBox (strict)"("Item Names"=string[] []) -> ()  [unwired: 2 in, 2 out]
        n157 = Reverse String(1:w387) -> (0:w386:string)
        n158 = Match Pattern(string=w386, regular expression=":") -> (before substring=w384:string, after substring=w383:string)  [unwired: 1 in, 2 out]
        n159 = local write "DCIR Profile"(waveform(dbl)[] [] ("EIS Profile")) -> ()
        n160 = local write "DCIR Nyquist"(cluster{dbl[], dbl[]} {[], []} ("EIS Nyquist")) -> ()
        n161 = Match Pattern(string=w383, regular expression="\\2E") -> (after substring=w381:string)  [unwired: 1 in, 3 out]
        n162 = Reverse String(1:w381) -> (0:w380:string)
        n163 = Reverse String(1:w384) -> (0:w379:string)
        n164 = Format Into String(format string="%s %s", w380, w379) -> (resulting string=w378:string)  [unwired: 2 in, 1 out]
        n165 = property class="VI"("Front Panel.Title"=w378) -> ()  [unwired: 2 in, 2 out]
        n166 = property on="Save DCIR Report" class="Bool"("DisabledEnum"=T6."Disabled and Grayed Out" ("Disabled")) -> ()  [unwired: 2 in, 2 out]
      }
      frame "UI: Cleanup" {
        n167 = property class="VI"() -> (error out=w394:errorcluster, "FP.State"=w396:T8)  [unwired: 2 in, 1 out]
        n168 = case shown="\"Standard\", Default" w396 {
          frame "Closed" {
          }
          frame "Standard", Default {
            n169 = invoke class="VI" method="FP.Close"() -> ()  [unwired: 3 in, 3 out]
          }
        }
      }
      frame "---------- CMD ----------" {
      }
      frame "CMD: Exit" {
      }
      frame "CMD: Front Panel State" {
        n170 = Format Into String(format string="UI: Front Panel State>>%s" ("string"), w405) -> (resulting string=w404:string)  [unwired: 2 in, 1 out]
        n171 = call <vilib>:"Add State(s) to Queue__jki_lib_state_machine.vi"("State(s) in (\"\")"=w408, "State(s) at Back (\"\")"=w404) -> ("States Out"=w407:string)  [unwired: 13 in]
      }
      frame "CMD: Start Profile" {
        n172 = Unbundle By Name(w416) -> ("Profile Complete Event"=w419:refnum<user-event>, "Core.Data"=w420:variant)
        n173 = call <vilib>:"Add State(s) to Queue__jki_lib_state_machine.vi"("State(s) in Front (\"\")"="DCIR: Start Profile", "State(s) in (\"\")"=w413) -> ("States Out"=w412:string)  [unwired: 13 in]
        n174 = Variant To Data(error in=w418, type=w419, Variant=w420) -> (data=w414:refnum<user-event>, error out=w417:errorcluster)
        n175 = Bundle By Name(cluster=w416, "Profile Complete Event"=w414) -> (w415:T3)
      }
      frame "CMD: Generate Plots" {
        n176 = call <vilib>:"Add State(s) to Queue__jki_lib_state_machine.vi"("State(s) in Front (\"\")"="DCIR: Generate Plots", "State(s) in (\"\")"=w423) -> ("States Out"=w422:string)  [unwired: 13 in]
      }
      frame "CMD: Stop Profile" {
        n177 = call <vilib>:"Add State(s) to Queue__jki_lib_state_machine.vi"("State(s) in Front (\"\")"="DCIR: Stop Profile", "State(s) in (\"\")"=w427) -> ("States Out"=w426:string)  [unwired: 13 in]
      }
    }
  }
  "error out" <- w4
  "reference out" <- "reference in"
